vi "Front Wheel Sensors.vi"(8 "Reset":bool, 9 "0 constant outside loop":i32, 11 "Input":bool) -> (3 "Output":i32)   [LabVIEW 2015]
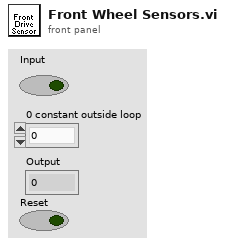
[diagram p1: front panel]
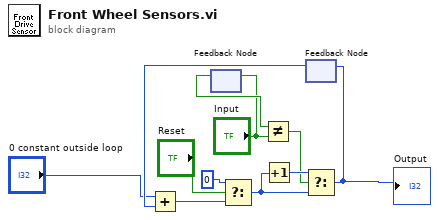
[diagram p0: block diagram]
diagram:
  n1 = feedback #1() -> (w10:bool)  [unwired: 1 in]
  n2 = feedback-in #1("Input") -> ()
  n3 = Not Equal?(x=w10, y="Input") -> (x != y?=w9:bool)
  n4 = feedback #2() -> (w8:i32)  [unwired: 1 in]
  n5 = Add(x="0 constant outside loop", y=w8) -> (x+y=w7:i32)
  n6 = Select(t=0, s="Reset", f=w7) -> (s? t:f=w6:i32)
  n7 = Increment(x=w6) -> (x+1=w11:i32)
  n8 = Select(t=w11, s=w9, f=w6) -> (s? t:f=w1:i32)
  "Output" <- w1
  n9 = feedback-in #2(w1) -> ()
